vi "g_average-of-waveform.vi"(1 "element":waveform(dbl)) -> (0 "array average":dbl)   [LabVIEW 2014]
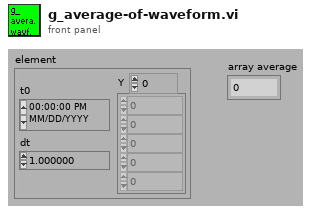
[diagram p1: front panel]
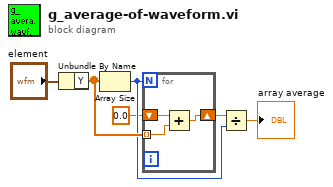
[diagram p0: block diagram]
diagram:
  n1 = Unbundle By Name("element") -> ("Y"=w6:dbl[])
  n2 = Array Size(array=w6) -> (size(s)=w4:i32)
  n3 = for {
    N: w4 -> [_]
    tunnel: w6 -> [w9] mode=indexing
    shift-right: [w8] -> w5
    shift-left: 0.0 -> [w7]
    n4 = Add(x=w7, y=w9) -> (x+y=w8:dbl)
  }
  n5 = Divide(x=w5, y=w4) -> (x/y=→"array average":dbl)
